vi "Place Trace Marker.vi"(8 "error in (no error)":errorcluster, 10 "Trace Marker":T1, 11 "SequenceViewPanel in":refnum<class "SequenceViewPanel.lvclass">) -> (0 "error out":errorcluster, 3 "SequenceViewPanel out":refnum<class "SequenceViewPanel.lvclass">)   [LabVIEW 2020, in "TSnax UI.lvlib" / "SequenceViewPanel.lvclass"]
uses:
  SequenceViewPanel.lvclass
  Trace Marker.ctl
  TSnax/SequenceFile/SequenceFile.lvclass
  SequenceViewPanel.lvclass/SequenceViewPanel.ctl
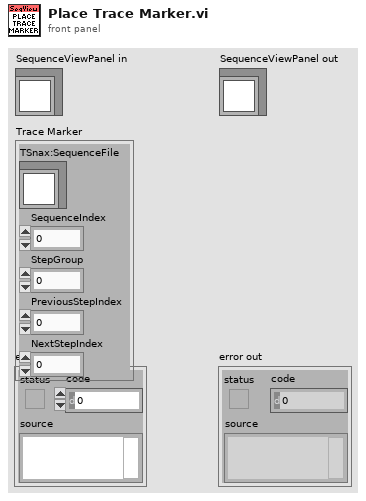
[diagram p1: front panel]
types:
  T1 = typedef "TSnax UI.lvlib/SequenceViewPanel.lvclass/Trace Marker.ctl" = cluster{"TSnax:SequenceFile":refnum<class "SequenceFile.lvclass">, "SequenceIndex":i32, "StepGroup":i32, "PreviousStepIndex":i32, "NextStepIndex":i32}
  T2 = typedef "TSnax UI.lvlib/SequenceViewPanel.lvclass/Ref Data.ctl" = cluster{"Insert Line":i32, "SequenceFile":refnum<class "SequenceFile.lvclass">, "Sequence":string, "Trace Marker":i32}
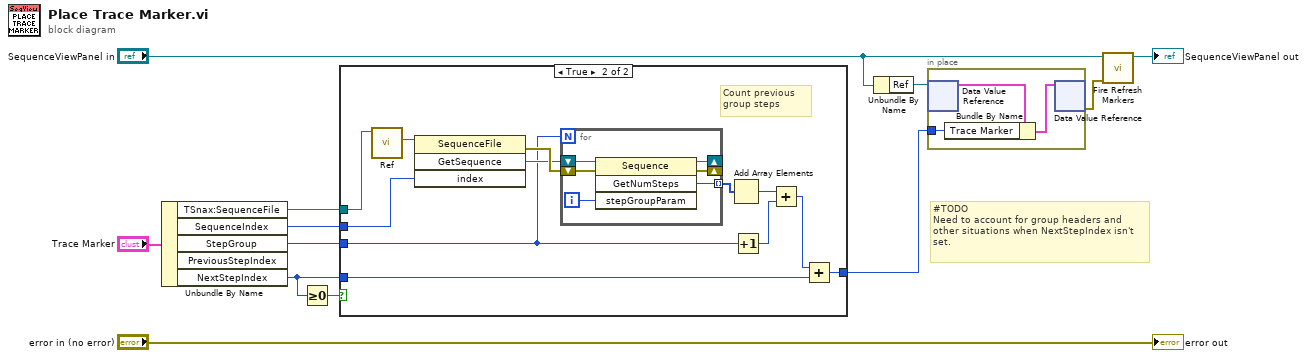
[diagram p0: block diagram]
diagram:
  # "#TODO\nNeed to account for group headers and other situations when NextStepIndex isn't set."
  n1 = Unbundle By Name("Trace Marker") -> ("TSnax:SequenceFile"=w10:refnum<class "SequenceFile.lvclass">, "SequenceIndex"=w9:i32, "StepGroup"=w8:i32, "NextStepIndex"=w2:i32)  [unwired: 1 out]
  n2 = Greater Or Equal To 0?(x=w2) -> (x >= 0?=w1:bool)
  n3 = case shown="True" w1 {
    tunnel: w10 -> [_ w24]
    tunnel: w9 -> [_ w22]
    tunnel: w8 -> [_ w18]
    tunnel: w2 -> [w13 w16]
    tunnel: [w13 w15] -> w6
    frame False {
    }
    frame True {
      # "Count previous group steps"
      n4 = call "Ref.vi"("SequenceFile in"=w24) -> ("Ref"=w23:refnum<k7>)  [unwired: 8 in, 2 out]
      n5 = invoke class="SequenceFile" method="GetSequence"(reference=w23, "index"=w22) -> (error out=w25:errorcluster, "GetSequence"=w21:refnum<k7>)  [unwired: 2 in, 2 out]
      n6 = for {
        N: w18 -> [_]
        shift-right: [w28] -> _
        shift-left: w25 -> [w31]
        shift-right: [w29] -> _
        shift-left: w21 -> [w30]
        tunnel: [w26] -> w20 mode=indexing
        i -> [w27]
        n7 = invoke class="Sequence" method="GetNumSteps"(reference=w30, error in=w31, "stepGroupParam"=w27) -> (reference out=w29:refnum<k7>, error out=w28:errorcluster, "GetNumSteps"=w26:i32)  [unwired: 1 in, 1 out]
      }
      n8 = Add Array Elements(numeric array=w20) -> (sum=w19:i32)
      n9 = Increment(x=w18) -> (x+1=w14:i32)
      n10 = Add(x=w19, y=w14) -> (x+y=w17:i32)
      n11 = Add(x=w17, y=w16) -> (x+y=w15:i32)
    }
  }
  n12 = Unbundle By Name("SequenceViewPanel in") -> ("Ref"=w7:refnum<data-value>)
  n13 = in-place {
    in-place-border: w6 -> [w32]
    n14 = in-place-dvr #1(w7) -> (w34:T2)  [unwired: 1 out]
    n15 = Bundle By Name(cluster=w34, "Trace Marker"=w32) -> (w33:T2)
    n16 = in-place-dvr #1(w33) -> (w3:errorcluster)  [unwired: 1 out]
  }
  n17 = call "Fire Refresh Markers.vi"("error in (no error)"=w3, "SequenceViewPanel in"="SequenceViewPanel in") -> ("SequenceViewPanel out"=→"SequenceViewPanel out":refnum<class "SequenceViewPanel.lvclass">)  [unwired: 8 in, 1 out]
  "error out" <- "error in (no error)"
